vi "ToString.vi"(8 "error in (no error)":errorcluster, 11 "IsFalse in":refnum<class "IsFalse.lvclass">) -> (0 "error out":errorcluster, 2 "String":string, 3 "IsFalse out":refnum<class "IsFalse.lvclass">)   [LabVIEW 2017, in "Transparent Assertions.lvlib" / "Constraints.lvlib" / "IsFalse.lvclass"]
doc: "Returns a string representation of the object."
uses:
  IsFalse.lvclass
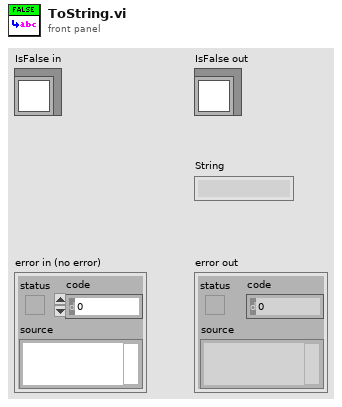
[diagram p1: front panel]
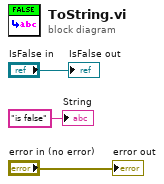
[diagram p0: block diagram]
diagram:
  "error out" <- "error in (no error)"
  "IsFalse out" <- "IsFalse in"
  "String" <- "is false" ("String")
